vi "FPGA_Temp.vi"() -> (2 "temp history":i16[](array[numeric]), 3 "Chassis Temperature":i16)   [LabVIEW 2020]
uses:
  <vilib>/rvi/Emulation/niFpgaGetClockAttributes.vi
  <vilib>/rvi/Emulation/niFpgaSctlEmulationGetInTimedLoop.vi
  <vilib>/rvi/Emulation/niFpgaEmulationReportErrorSimple.vi
  <vilib>/rvi/eio/common/nirviEmuTemplateMethod_errors.vi
  <vilib>/rvi/Emulation/niFpgaCriticalErrorInLSC.vi
  <vilib>/eio/EIONode/EIONode.xnode
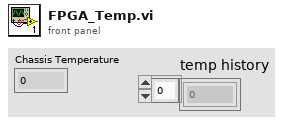
[diagram p1: front panel]
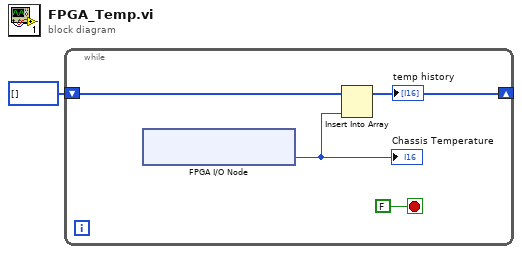
[diagram p0: block diagram]
diagram:
  n1 = while {
    shift-right: [w3] -> _
    shift-left: i16[] [] -> [w2]
    stop <- FALSE stop-if-true
    n2 = xnode "FPGA I/O Node"() -> ("Chassis Temperature"=w4:i16)  [unwired: 1 in, 1 out]
    "Chassis Temperature" <- w4
    n3 = Insert Into Array(array=w2, new element=w4) -> (w3:i16[])  [unwired: 1 in]
    "temp history" <- w3
  }
